vi "Python_example.vi"(10 "Numeric in":i32, 11 "module path":path) -> (3 "Numeric out":i32)   [LabVIEW 2020]
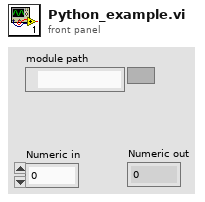
[diagram p1: front panel]
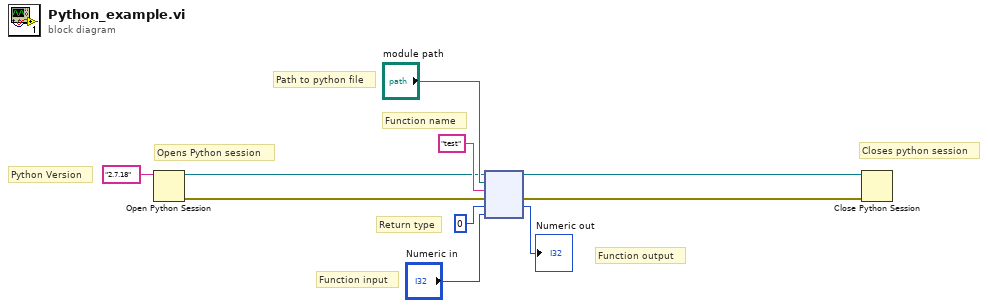
[diagram p0: block diagram]
diagram:
  # "Opens Python session"
  # "Closes python session"
  # "Function output"
  # "Function input"
  # "Return type"
  # "Path to python file"
  # "Function name"
  # "Python Version"
  n1 = Open Python Session(python version="2.7.18" ("Python version")) -> (session out=w1:refnum<k35>, error out=w4:errorcluster)  [unwired: 2 in]
  n2 = node(w1, "module path", "test" ("function name"), w4, 0 ("Numeric"), "Numeric in") -> (w2:refnum<k35>, w3:errorcluster, →"Numeric out":i32)  [unwired: 1 in, 2 out]
  n3 = Close Python Session(session in=w2, error in=w3) -> ()  [unwired: 1 out]
